vi "SaveHisto.vi"(2 "error in":errorcluster, 3 "Array":dbl[](array[numeric]), 4 "String":string, 5 "storage refnum (file)":refnum<k20>) -> (0 "error out":errorcluster, 1 "storage refnum (file) out":refnum<k20>)   [LabVIEW 2014]
uses:
  <vilib>/Platform/storage/Storage.llb/usiSequenceRepresentation.ctl
  <vilib>/Platform/storage/Storage.llb/usiOverwriteOptions.ctl
  <vilib>/Platform/storage/lvStorage.llb/_createOrGetByNameExplicitChildObject.vi
  <vilib>/Platform/storage/Storage.llb/__savePropString.vi
  <vilib>/Platform/storage/lvStorage.llb/xStorage/xStorageSupp/ErrorOut.vi
  <vilib>/Platform/storage/lvStorage.llb/_saveFloat64Channel.vi
  <vilib>/Platform/storage/lvStorage.llb/xStorage/Write Data/Write Data.xnode
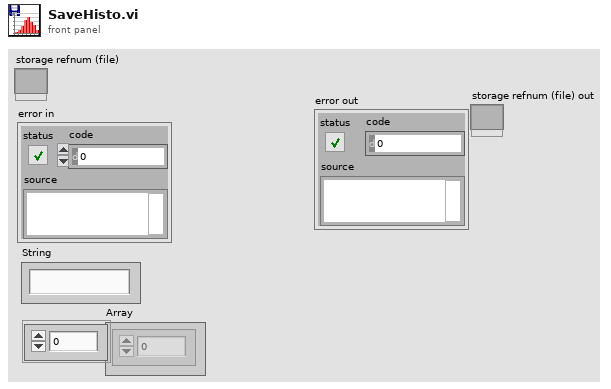
[diagram p1: front panel]
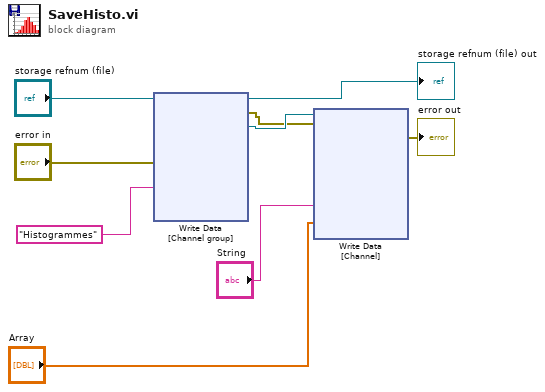
[diagram p0: block diagram]
diagram:
  n1 = xnode "Write Data\n[Channel group]"("Name"="Histogrammes", "storage refnum (file)"="storage refnum (file)", "error in"="error in") -> ("storage refnum (file) out"=→"storage refnum (file) out":refnum<k20>, "error out"=w7:errorcluster, "storage refnum (channel group)"=w8:refnum<k20>)  [unwired: 1 in]
  n2 = xnode "Write Data\n[Channel]"("Name"="String", "Signal"="Array", "storage refnum (channel group)"=w8, "error in"=w7) -> ("error out"=→"error out":errorcluster)  [unwired: 2 in, 2 out]
